vi "uPython_Comm.vi"(6 "FIFO Size":i32=100000, 7 "Wait for Reply?":bool, 8 "error in (no error)":errorcluster, 9 "Console In":string, 10 "Script":string, 11 "VISA Refnum in":refnum<visa-resource-name>) -> (0 "error out":errorcluster, 1 "Console Out":string, 2 "Buffer":string, 3 "VISA out":refnum<visa-resource-name>, 5 "Update?":bool)   [LabVIEW 2016]
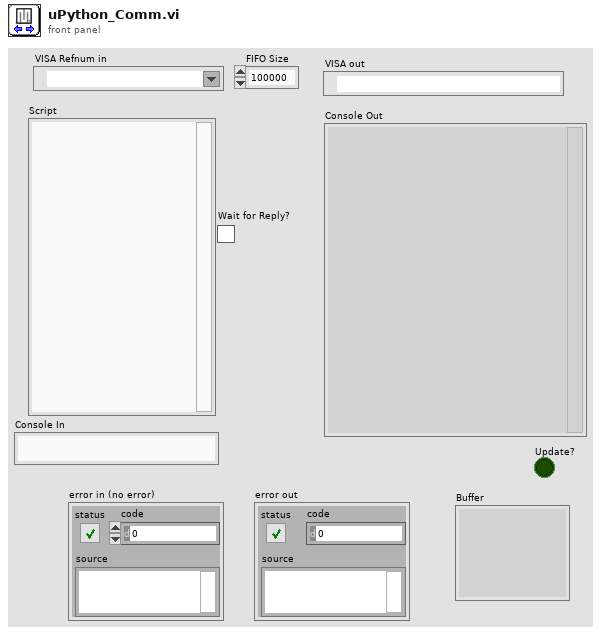
[diagram p1: front panel]
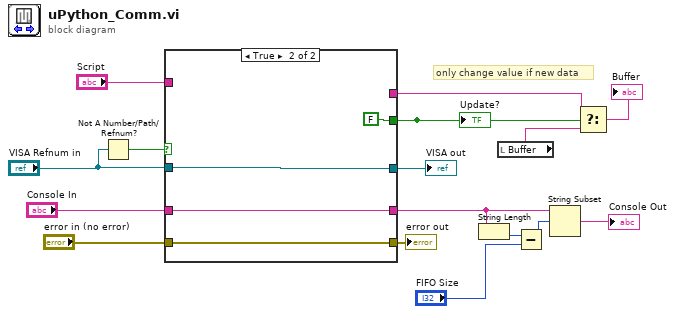
[diagram p0: block diagram]
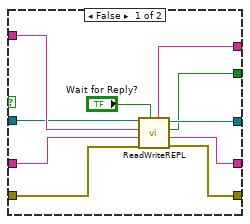
[diagram p2: hidden frame]
diagram:
  # "only change value if new data"
  n1 = Not A Number/Path/Refnum?(number/path/refnum="VISA Refnum in") -> (NaN/Path/Refnum?=w11:bool)
  n2 = case shown="True" w11 {
    tunnel: [w25 w30] -> w16
    tunnel: [w24 w29] -> w15
    tunnel: "Script" -> [w23 _]
    tunnel: "error in (no error)" -> [w19 w29]
    tunnel: "VISA Refnum in" -> [w18 w30]
    tunnel: [w26 w28] -> w6
    tunnel: "Console In" -> [w20 w28]
    tunnel: [w22 FALSE ("Update?")] -> w4
    tunnel: [w17 _] -> w3
    frame False {
      n3 = call <userlib>:"ReadWriteREPL.vi"("Wait?"="Wait for Reply?", "error in"=w19, "Console In"=w20, "write buffer"=w23, "VISA in"=w18) -> ("error out"=w24:errorcluster, "Console Out"=w26:string, "Update?"=w22:bool, "VISA out"=w25:refnum<visa-resource-name>, "new text"=w17:string)  [unwired: 2 in]
    }
    frame True {
    }
  }
  "VISA out" <- w16
  "error out" <- w15
  "Update?" <- w4
  n4 = String Length(string=w6) -> (length=w9:i32)
  n5 = local read "Buffer"() -> (w2:string)
  n6 = Subtract(x=w9, y="FIFO Size") -> (x-y=w7:i32)
  n7 = String Subset(string=w6, offset (0)=w7) -> (substring=→"Console Out":string)  [unwired: 1 in]
  n8 = Select(t=w3, s=w4, f=w2) -> (s? t:f=→"Buffer":string)
